vi "GetConfig.vi"(8 "error in (no error)":errorcluster, 11 "ArbitraryFunction in":refnum<class "ArbitraryFunction.lvclass">) -> (0 "error out":errorcluster, 2 "Config":variant, 3 "ArbitraryFunction out":refnum<class "ArbitraryFunction.lvclass">)   [LabVIEW 2018, in "Functions.lvlib" / "ArbitraryFunction.lvclass"]
uses:
  ArbitraryFunction.lvclass
  TypeDefs/ArbCfg.ctl
  TypeDefs/Arbitrary.ctl
  ArbitraryFunction.lvclass/ArbitraryFunction.ctl
  Accessors/Read Arbs.vi
  Accessors/Read SampleRate.vi
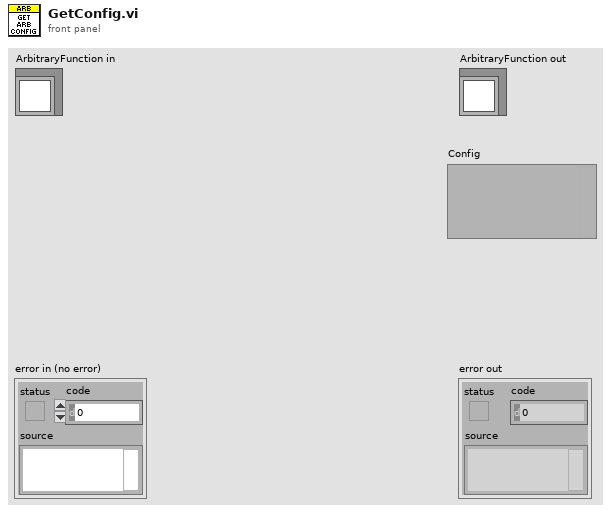
[diagram p1: front panel]
types:
  T1 = typedef "Functions.lvlib/ArbitraryFunction.lvclass/ArbCfg.ctl" = cluster{"SampleRate":dbl, "Count":u16, "Arbs":T2[]}
  T2 = typedef "Functions.lvlib/ArbitraryFunction.lvclass/Arbitrary.ctl" = cluster{"Handle":string, "Size":i32, "Gain":dbl, "Offset":dbl, "Waveform":waveform(dbl)}
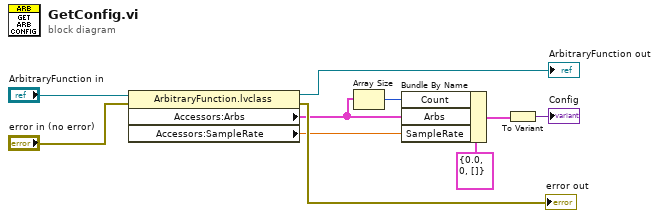
[diagram p0: block diagram]
diagram:
  n1 = property class="ArbitraryFunction.lvclass"(reference="ArbitraryFunction in", error in="error in (no error)") -> (reference out=→"ArbitraryFunction out":refnum<class "ArbitraryFunction.lvclass">, error out=→"error out":errorcluster, "Accessors:Arbs"=w3:T2[], "Accessors:SampleRate"=w2:dbl)
  n2 = Array Size(array=w3) -> (size(s)=w4:i32)
  n3 = Bundle By Name(cluster=T1 {"SampleRate"=0.0, "Count"=0, "Arbs"=[]} ("ArbCfg"), "Count"=w4, "Arbs"=w3, "SampleRate"=w2) -> (w1:T1)
  n4 = To Variant(anything=w1) -> (Variant=→"Config":variant)
